vi "GetSubSettingPath.vi"(10 "settings file name":string, 11 "LabVIEW Data Path":path) -> (3 "settings file path":path)   [LabVIEW 2022 SP3]
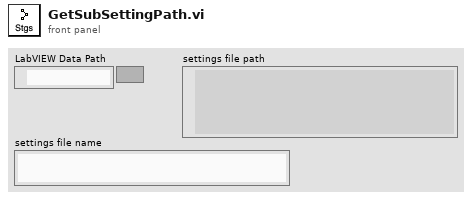
[diagram p1: front panel]
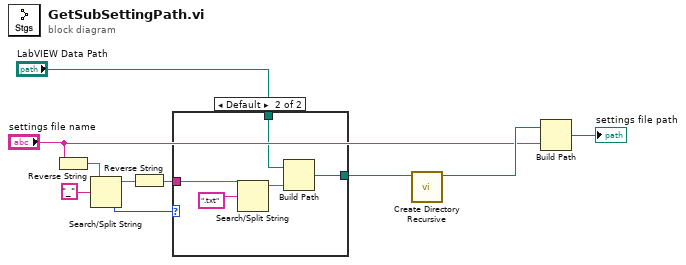
[diagram p0: block diagram]
diagram:
  n1 = Reverse String(1:"settings file name") -> (0:w5:string)
  n2 = Search/Split String(string=w5, search string/char (-)="_" ("y")) -> (substring before match=w7:string, offset of match=w6:i32)  [unwired: 1 in, 1 out]
  n3 = Reverse String(1:w7) -> (0:w8:string)
  n4 = case shown="Default" w6 {
    tunnel: w8 -> [_ w16]
    tunnel: "LabVIEW Data Path" -> [w11 w13]
    tunnel: [w11 w12] -> w9
    frame -1 {
    }
    frame Default {
      n5 = Search/Split String(string=w16, search string/char (-)=".txt" ("y")) -> (substring before match=w14:string)  [unwired: 1 in, 2 out]
      n6 = Build Path(base path=w13, name or relative path=w14) -> (appended path=w12:path)
    }
  }
  n7 = call <vilib>:"Create Directory Recursive.vi"("directory"=w9) -> ("directory copy"=w10:path)  [unwired: 4 in, 2 out]
  n8 = Build Path(base path=w10, name or relative path="settings file name") -> (appended path=→"settings file path":path)
